vi "VM_ProjetoV2.vi"() -> ()   [LabVIEW 2016]
uses:
  <vilib>/vision/NI_Vision_Development_Module.lvlib
panel:
  out "Image Out 2":T1(plugin-control)
  out "Image Out":T1(plugin-control)
  in  "Source":path=path "C:/Users/Alexandre/Documents/LabView Projects/Projeto/Source"
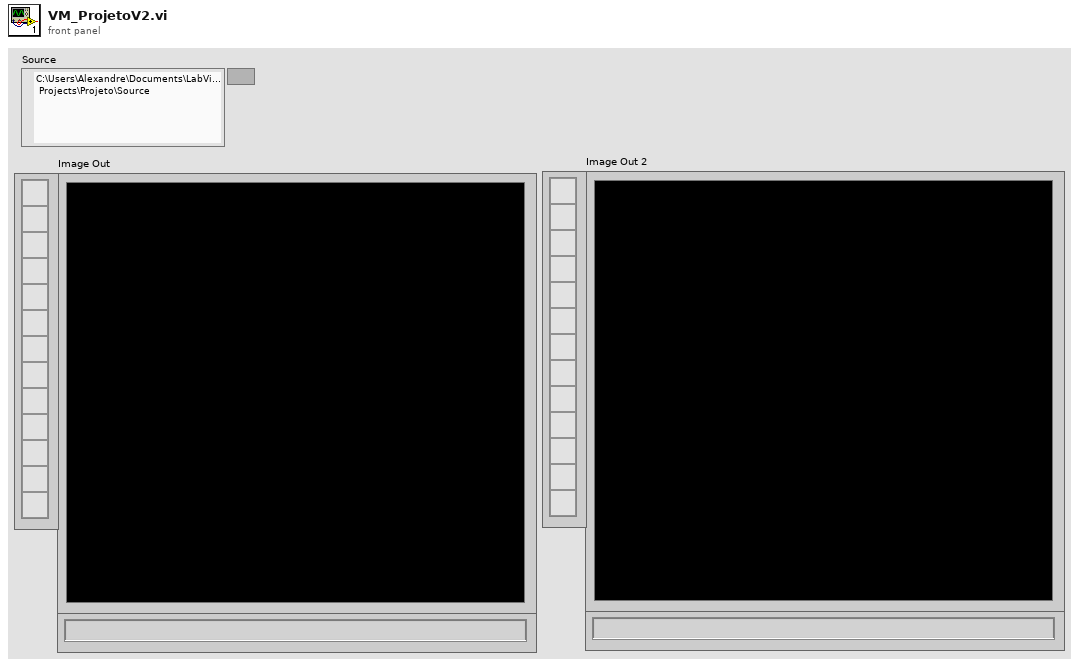
[diagram p1: front panel]
types:
  T1 = typedef "IMAQ Image.ctl" = refnum<image>
  T2 = cluster{"Position":cluster{"x":sgl, "y":sgl}, "Angle":sgl, "Scale":sgl, "Score":sgl, "Bounding Box":cluster{"x":sgl, "y":sgl}[]}[]
  T3 = typedef "IMAQ Rectangle" = cluster{"Left":i32, "Top":i32, "Right":i32, "Bottom":i32, "Rotation":dbl}
  T4 = typedef "ROI Descriptor" = cluster{"Global Rectangle":i32[], "Contours":cluster{"ID":enum32{"External", "Internal"}, "Type":u32, "Coordinates":i32[]}[]}
  T5 = typedef "Image Type" = u32
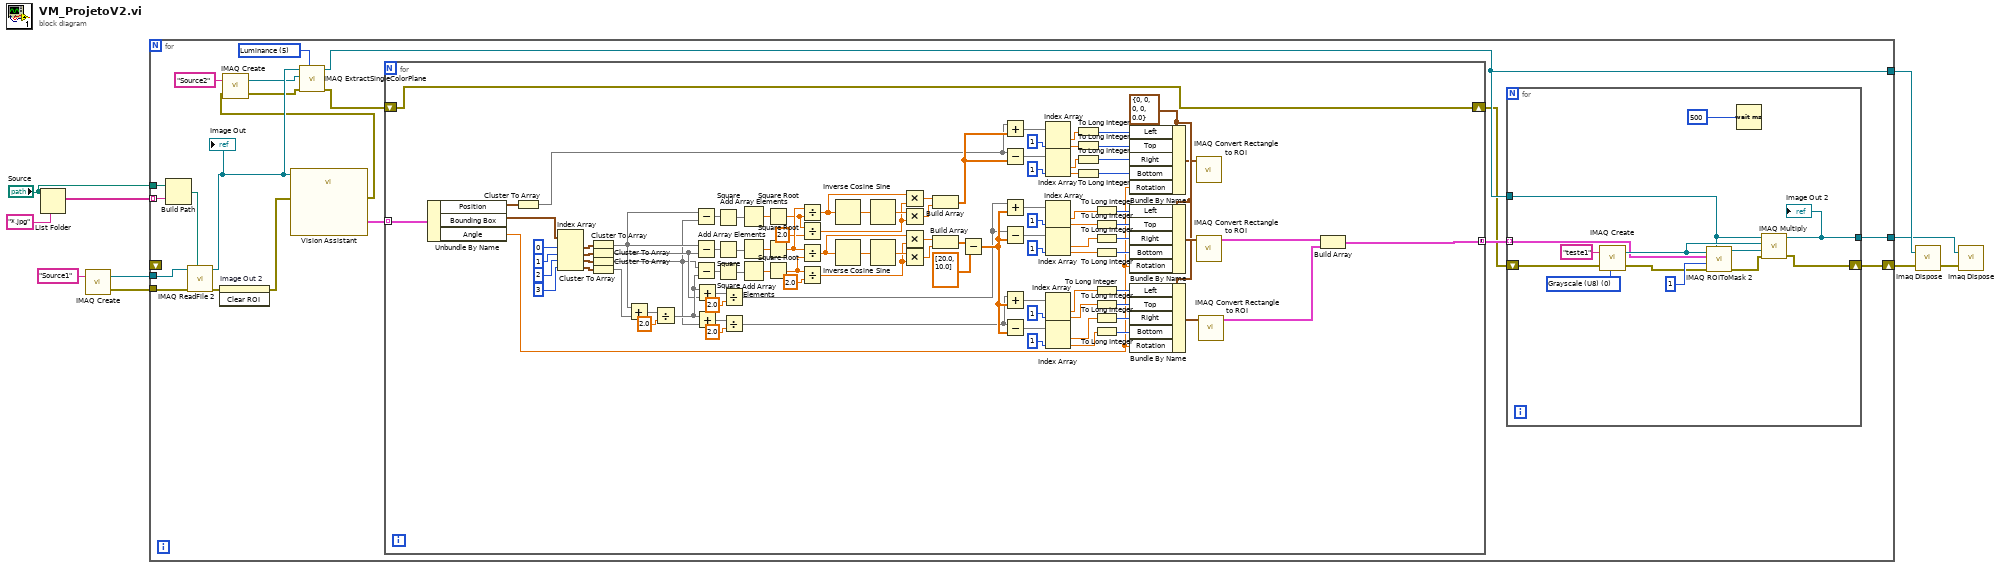
[diagram p0: block diagram]
diagram:
  n1 = List Folder(path="Source", pattern="*.jpg") -> (filenames=w9:string[])  [unwired: 2 in, 3 out]
  n2 = call "IMAQ Create"("Image Name"="Source1") -> ("New Image"=w6:T1, "error out"=w5:errorcluster)  [unwired: 4 in]
  n3 = for {
    tunnel: w9 -> [w30] mode=indexing
    tunnel: "Source" -> [w29]
    tunnel: w6 -> [w28]
    tunnel: w5 -> [w27]
    shift-right: [w18] -> w4
    shift-left: _ -> [_]
    tunnel: [w16] -> w3
    tunnel: [w17] -> w1
    w20 = 5 items=["Red", "Green", "Blue", "Hue", "Saturation", "Luminance", "Value", "Intensity"] ("Color Plane")
    n4 = Build Path(base path=w29, name or relative path=w30) -> (appended path=w26:path)
    n5 = call "IMAQ ReadFile 2"("File Path"=w26, "error in (no error)"=w27, "Image"=w28) -> ("error out"=w24:errorcluster, "Image Out"=w23:T1)  [unwired: 4 in, 3 out]
    "Image Out" <- w23
    n6 = invoke on="Image Out 2" class="ImageControl" method="Clear ROI"(error in=w24) -> (error out=w19:errorcluster)  [unwired: 2 in, 2 out]
    n7 = call "Vision Assistant"("Image In"=w23, "error in"=w19) -> ("Matches (Pattern Matching 1)"=w25:T2, "error out"=w14:errorcluster)  [unwired: 23 in, 1 out]
    n8 = call "IMAQ Create"("Image Name"="Source2", "error in (no error)"=w14) -> ("New Image"=w21:T1, "error out"=w13:errorcluster)  [unwired: 3 in]
    n9 = call "IMAQ ExtractSingleColorPlane"("Color Plane"=w20, "error in (no error)"=w13, "Image Dst"=w21, "Image Src"=w23) -> ("error out"=w12:errorcluster, "Image Dst Out"=w16:T1)  [unwired: 6 in]
    n10 = for {
      tunnel: w25 -> [w143] mode=indexing
      tunnel: [w50] -> w15 mode=concatenating
      shift-right: [w44] -> w11
      shift-left: w12 -> [w44]
      w63 = T3 {"Left"=0, "Top"=0, "Right"=0, "Bottom"=0, "Rotation"=0.0} ("Rectangle")
      n11 = Unbundle By Name(w143) -> ("Position"=w53:cluster{"x":sgl, "y":sgl}, "Bounding Box"=w84:cluster{"x":sgl, "y":sgl}[], "Angle"=w49:sgl)
      n12 = Cluster To Array(cluster=w53) -> (array=w52:sgl[])
      n13 = Index Array(array=w84, index #1=0 ("index"), index #2=1 ("index"), index #3=2 ("index"), index #4=3 ("index")) -> (element #1=w142:cluster{"x":sgl, "y":sgl}, element #2=w141:cluster{"x":sgl, "y":sgl}, element #3=w140:cluster{"x":sgl, "y":sgl}, element #4=w139:cluster{"x":sgl, "y":sgl})
      n14 = Cluster To Array(cluster=w142) -> (array=w74:sgl[])
      n15 = Cluster To Array(cluster=w141) -> (array=w124:sgl[])
      n16 = Cluster To Array(cluster=w140) -> (array=w73:sgl[])
      n17 = Cluster To Array(cluster=w139) -> (array=w138:sgl[])
      n18 = Add(x=w74, y=w138) -> (x+y=w137:sgl[])
      n19 = Divide(x=w137, y=sgl 2.0) -> (x/y=w125:sgl[])
      n20 = Subtract(x=w74, y=w73) -> (x-y=w77:sgl[])
      n21 = Subtract(x=w74, y=w124) -> (x-y=w133:sgl[])
      n22 = Subtract(x=w73, y=w125) -> (x-y=w132:sgl[])
      n23 = Add(x=w125, y=w124) -> (x+y=w129:sgl[])
      n24 = Add(x=w125, y=w73) -> (x+y=w126:sgl[])
      n25 = Square(x=w77) -> (x^2=w76:sgl[])
      n26 = Square(x=w133) -> (x^2=w134:sgl[])
      n27 = Square(x=w132) -> (x^2=w131:sgl[])
      n28 = Divide(x=w129, y=sgl 2.0) -> (x/y=w79:sgl[])
      n29 = Divide(x=w126, y=sgl 2.0) -> (x/y=w78:sgl[])
      n30 = Add Array Elements(numeric array=w76) -> (sum=w75:sgl)
      n31 = Add Array Elements(numeric array=w134) -> (sum=w135:sgl)
      n32 = Add Array Elements(numeric array=w131) -> (sum=w130:sgl)
      n33 = Square Root(x=w75) -> (sqrt(x)=w68:sgl)
      n34 = Square Root(x=w135) -> (sqrt(x)=w72:sgl)
      n35 = Square Root(x=w130) -> (sqrt(x)=w121:sgl)
      n36 = Divide(x=w72, y=w68) -> (x/y=w67:sgl)
      n37 = Divide(x=w68, y=sgl 2.0) -> (x/y=w66:sgl)
      n38 = Divide(x=w72, y=w121) -> (x/y=w117:sgl)
      n39 = Divide(x=w121, y=sgl 2.0) -> (x/y=w116:sgl)
      n40 = Inverse Cosine(1:w67) -> (0:w71:sgl)
      n41 = Inverse Cosine(1:w117) -> (0:w123:sgl)
      n42 = Sine(x=w71) -> (sin(x)=w70:sgl)
      n43 = Sine(x=w123) -> (sin(x)=w118:sgl)
      n44 = Multiply(x=w67, y=w66) -> (x*y=w64:sgl)
      n45 = Multiply(x=w70, y=w66) -> (x*y=w65:sgl)
      n46 = Multiply(x=w117, y=w116) -> (x*y=w119:sgl)
      n47 = Multiply(x=w118, y=w116) -> (x*y=w120:sgl)
      n48 = Build Array(w64, w65) -> (w54:sgl[])
      n49 = Build Array(w119, w120) -> (w87:sgl[])
      n50 = Subtract(x=w87, y=sgl[] [20.0, 10.0]) -> (x-y=w86:sgl[])
      n51 = Add(x=w52, y=w54) -> (x+y=w62:sgl[])
      n52 = Subtract(x=w52, y=w54) -> (x-y=w59:sgl[])
      n53 = Add(x=w79, y=w86) -> (x+y=w103:sgl[])
      n54 = Subtract(x=w79, y=w86) -> (x-y=w106:sgl[])
      n55 = Add(x=w78, y=w86) -> (x+y=w102:sgl[])
      n56 = Subtract(x=w78, y=w86) -> (x-y=w99:sgl[])
      n57 = Index Array(array=w62, index #2=1 ("index")) -> (element #1=w58:sgl, element #2=w57:sgl)  [unwired: 1 in]
      n58 = Index Array(array=w59, index #2=1 ("index")) -> (element #1=w56:sgl, element #2=w55:sgl)  [unwired: 1 in]
      n59 = Index Array(array=w103, index #2=1 ("index")) -> (element #1=w111:sgl, element #2=w112:sgl)  [unwired: 1 in]
      n60 = Index Array(array=w106, index #2=1 ("index")) -> (element #1=w113:sgl, element #2=w114:sgl)  [unwired: 1 in]
      n61 = Index Array(array=w102, index #2=1 ("index")) -> (element #1=w94:sgl, element #2=w93:sgl)  [unwired: 1 in]
      n62 = Index Array(array=w99, index #2=1 ("index")) -> (element #1=w92:sgl, element #2=w91:sgl)  [unwired: 1 in]
      n63 = To Long Integer(number=w58) -> (32bit integer=w48:i32)
      n64 = To Long Integer(number=w57) -> (32bit integer=w47:i32)
      n65 = To Long Integer(number=w56) -> (32bit integer=w46:i32)
      n66 = To Long Integer(number=w55) -> (32bit integer=w45:i32)
      n67 = To Long Integer(number=w111) -> (32bit integer=w107:i32)
      n68 = To Long Integer(number=w112) -> (32bit integer=w108:i32)
      n69 = To Long Integer(number=w113) -> (32bit integer=w109:i32)
      n70 = To Long Integer(number=w114) -> (32bit integer=w110:i32)
      n71 = To Long Integer(number=w94) -> (32bit integer=w98:i32)
      n72 = To Long Integer(number=w93) -> (32bit integer=w97:i32)
      n73 = To Long Integer(number=w92) -> (32bit integer=w96:i32)
      n74 = To Long Integer(number=w91) -> (32bit integer=w95:i32)
      n75 = Bundle By Name(cluster=w63, "Left"=w48, "Top"=w47, "Right"=w46, "Bottom"=w45, "Rotation"=w49) -> (w51:T3)
      n76 = Bundle By Name(cluster=w63, "Left"=w107, "Top"=w108, "Right"=w109, "Bottom"=w110, "Rotation"=w49) -> (w115:T3)
      n77 = Bundle By Name(cluster=w63, "Left"=w98, "Top"=w97, "Right"=w96, "Bottom"=w95, "Rotation"=w49) -> (w90:T3)
      n78 = call "IMAQ Convert Rectangle to ROI"("Rectangle"=w51) -> ()  [unwired: 8 in, 2 out]
      n79 = call "IMAQ Convert Rectangle to ROI"("Rectangle"=w115) -> ("ROI Descriptor"=w89:T4)  [unwired: 8 in, 1 out]
      n80 = call "IMAQ Convert Rectangle to ROI"("Rectangle"=w90) -> ("ROI Descriptor"=w88:T4)  [unwired: 8 in, 1 out]
      n81 = Build Array(w89, w88) -> (w50:T4[])
    }
    n82 = for {
      tunnel: w16 -> [w36]
      shift-right: [w34] -> w18
      shift-left: w11 -> [w35]
      tunnel: [w33] -> w17
      tunnel: w15 -> [w31] mode=indexing
      w41 = T5 0 items=["Grayscale (U8)", "Grayscale (I16)", "Grayscale (SGL)", "Complex (CSG)", "RGB (U32)", "HSL (U32)", "RGB (U64)", "Grayscale (U16)"] ("Image Type")
      n83 = call "IMAQ Create"("Image Name"="teste1", "Image Type"=w41, "error in (no error)"=w35) -> ("New Image"=w37:T1, "error out"=w38:errorcluster)  [unwired: 2 in]
      n84 = call "IMAQ ROIToMask 2"("Image Model"=w36, "error in (no error)"=w38, "Filling Value (255)"=1, "ROI Descriptor"=w31, "Image"=w37) -> ("error out"=w43:errorcluster, "Image Out"=w40:T1)  [unwired: 4 in, 1 out]
      n85 = Wait (ms)(milliseconds to wait=u32 500 ("millisecond multiple")) -> ()  [unwired: 1 out]
      n86 = call "IMAQ Multiply"("Image Src A"=w36, "Image Dst"=w37, "Image Src B"=w40, "error in (no error)"=w43) -> ("Image Dst Out"=w33:T1, "error out"=w34:errorcluster)  [unwired: 3 in]
      "Image Out 2" <- w33
    }
  }
  n87 = call "Imaq Dispose"("Image"=w3, "error in (no error)"=w4) -> ("error out"=w2:errorcluster)  [unwired: 4 in]
  n88 = call "Imaq Dispose"("Image"=w1, "error in (no error)"=w2) -> ()  [unwired: 4 in, 1 out]
